vi "Destroy User Events.vi"(11 "Host MSS Test Actor in":refnum<class "Host MSS Test Actor.lvclass">) -> (3 "Host MSS Test Actor out":refnum<class "Host MSS Test Actor.lvclass">)   [LabVIEW 2023, in "Host MSS Test Actor.lvlib" / "Host MSS Test Actor.lvclass"]
uses:
  Host MSS Test Actor.lvclass
  Host MSS Test Actor.lvclass/Host MSS Test Actor.ctl
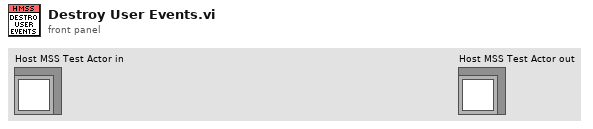
[diagram p1: front panel]
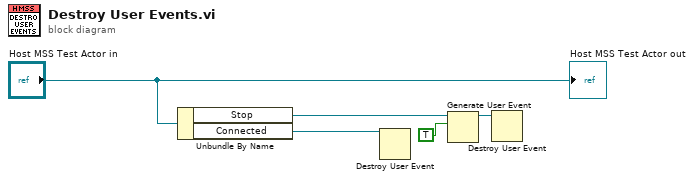
[diagram p0: block diagram]
diagram:
  n1 = Unbundle By Name("Host MSS Test Actor in") -> ("Stop"=w3:refnum<user-event>, "Connected"=w4:refnum<user-event>)
  n2 = Destroy User Event(user event=w4) -> ()  [unwired: 1 in, 1 out]
  n3 = Generate User Event(user event=w3, event data cluster=TRUE ("event data")) -> (user event out=w2:refnum<user-event>)  [unwired: 2 in, 1 out]
  n4 = Destroy User Event(user event=w2) -> ()  [unwired: 1 in, 1 out]
  "Host MSS Test Actor out" <- "Host MSS Test Actor in"
